vi "M300ShiftRun.vi"() -> ()   [LabVIEW 2012]
uses:
  <vilib>/Utility/miscctls.llb/LVDateTimeRec.ctl
panel:
  out "array":string[][](array[string])
  out "date string 2":string
  out "EndTime 3":string
  out "EndTime 2":string
  out "Numeric":i32
  out "date string 3":string
  out "©]1-4":dbl
  out "©]1-3":dbl
  out "早1-1":dbl
  out "©]1-1":dbl
  out "©]1-2":dbl
  out "早1-2":dbl
  out "©]2":dbl
  out "早2":dbl
  out "©]1":dbl
  out "早1":dbl
  in  "stop":bool
  out "中2":dbl
  out "中班1":dbl
  out "Start":timestamp
  out "End":timestamp
  out "ShiftC":timestamp
  out "ShiftA":timestamp
  out "ShiftB":timestamp
  out "date string":string
  out "x/y":dbl
  out "date/time string 2":string
  out "date/time string":string
  in  "EndTime":string
  in  "EndDate":string
  in  "BegTime":string
  in  "BegDate":string
  in  "date time rec":T1
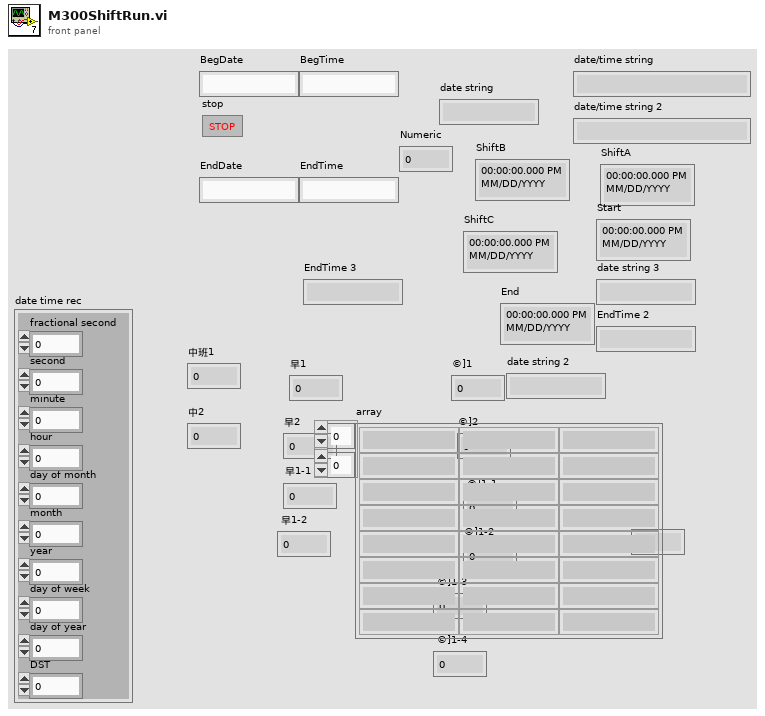
[diagram p1: front panel]
types:
  T1 = typedef "LVDateTimeRec.ctl" = cluster{"fractional second":dbl, "second":i32, "minute":i32, "hour":i32, "day of month":i32, "month":i32, "year":i32, "day of week":i32, "day of year":i32, "DST":i32}
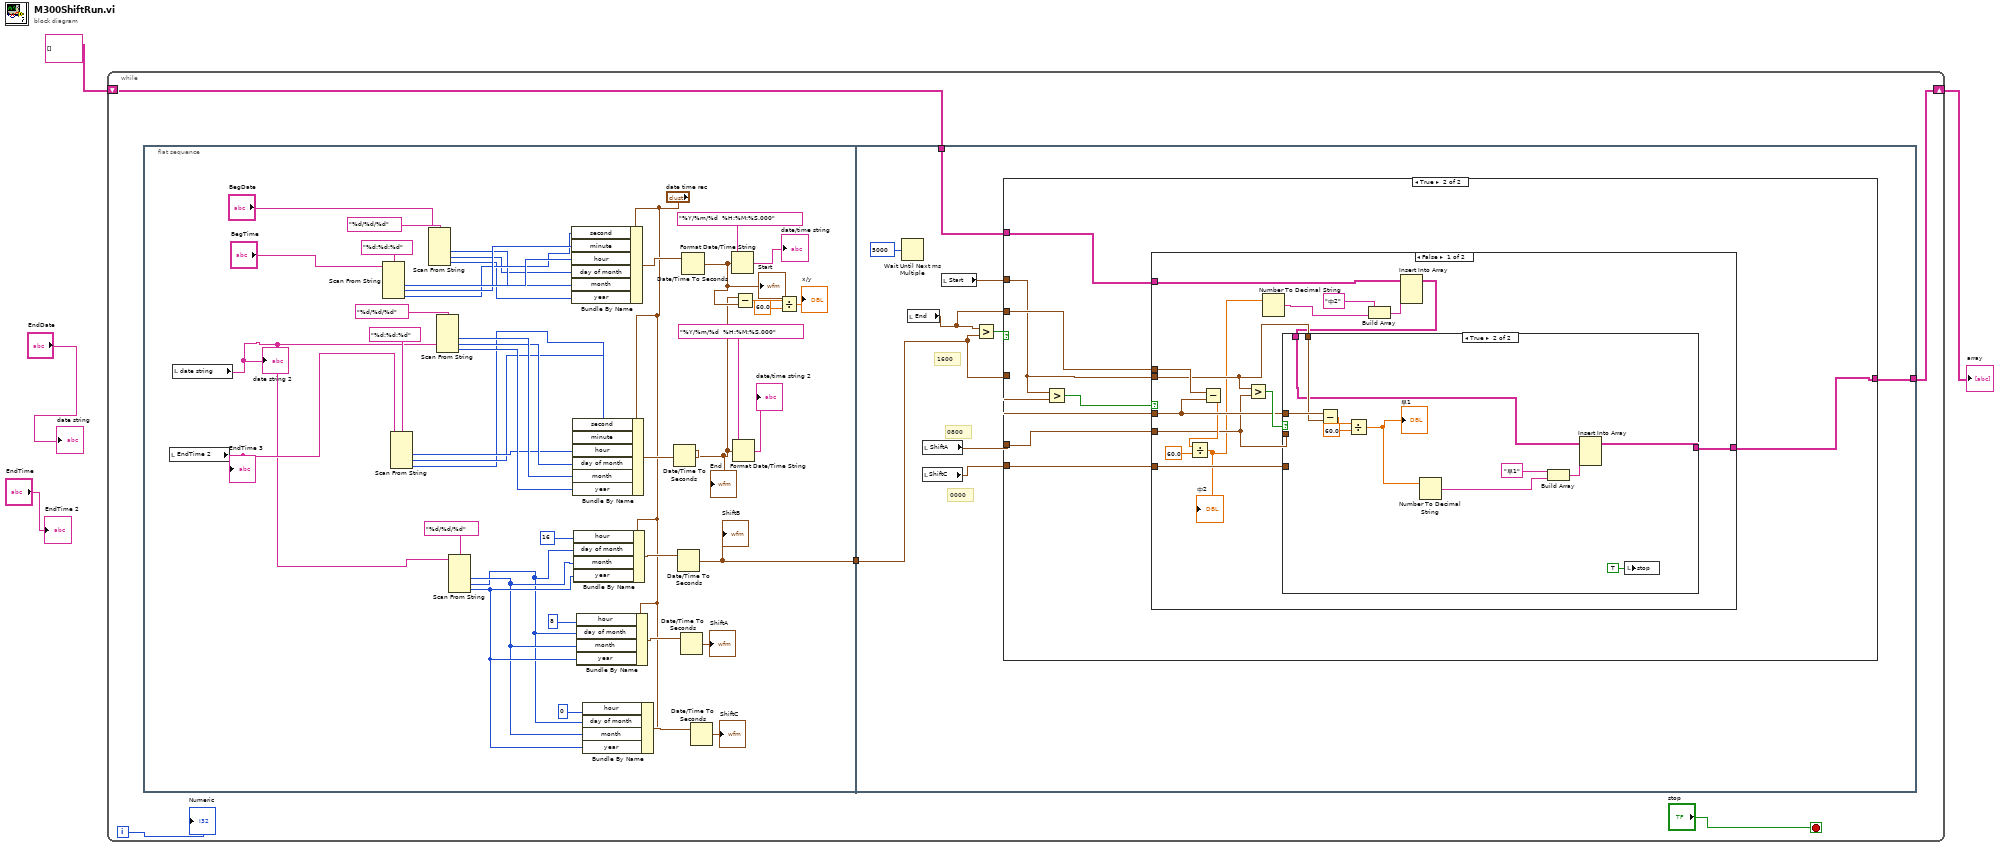
[diagram p0: block diagram]
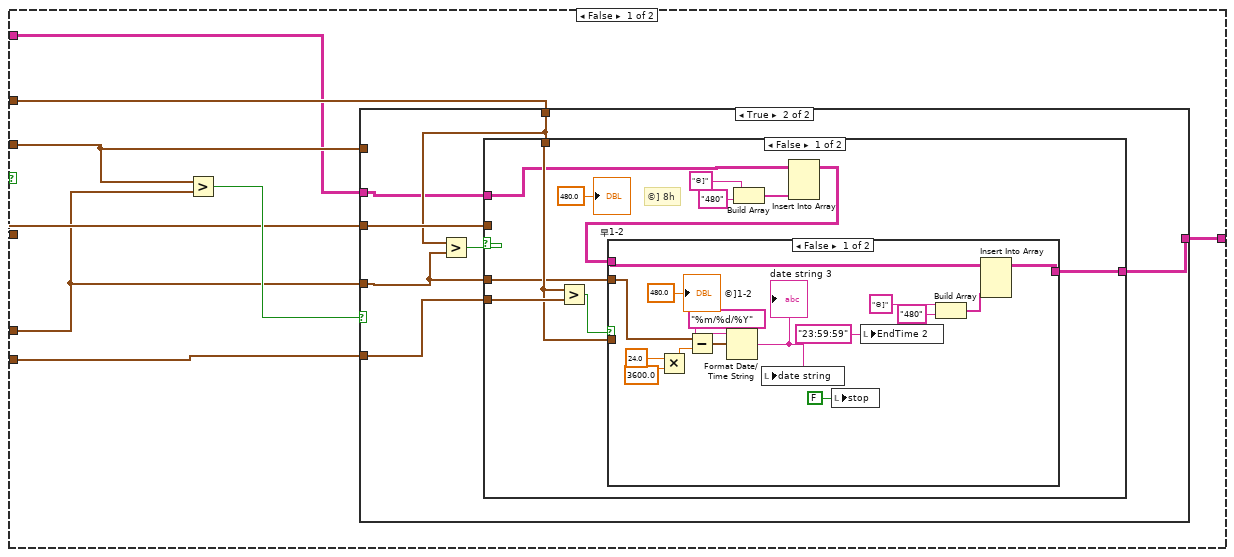
[diagram p2: hidden frame]
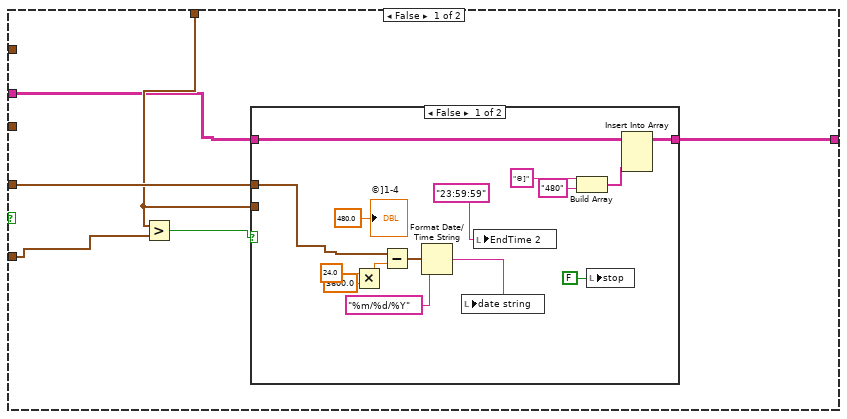
[diagram p3: hidden frame]
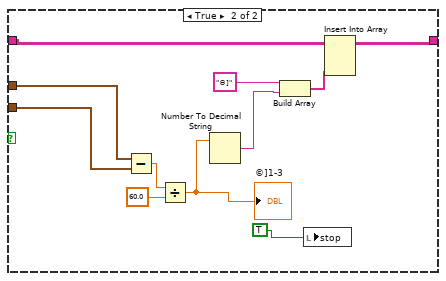
[diagram p4: hidden frame]
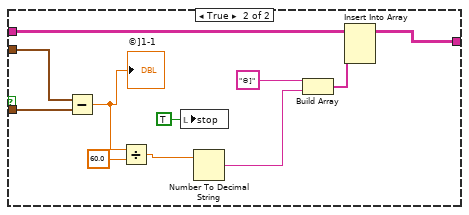
[diagram p5: hidden frame]
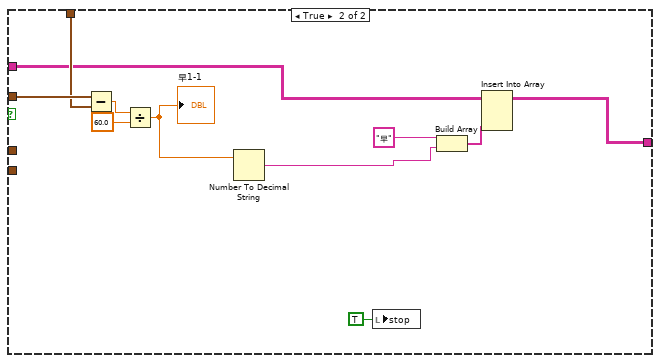
[diagram p6: hidden frame]
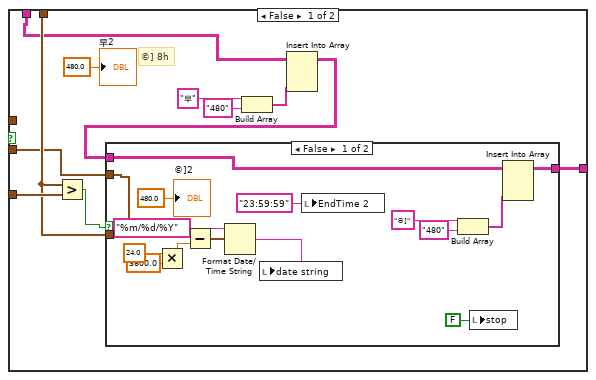
[diagram p7: hidden frame]
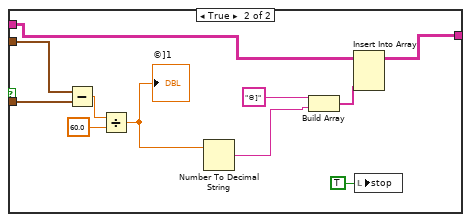
[diagram p8: hidden frame]
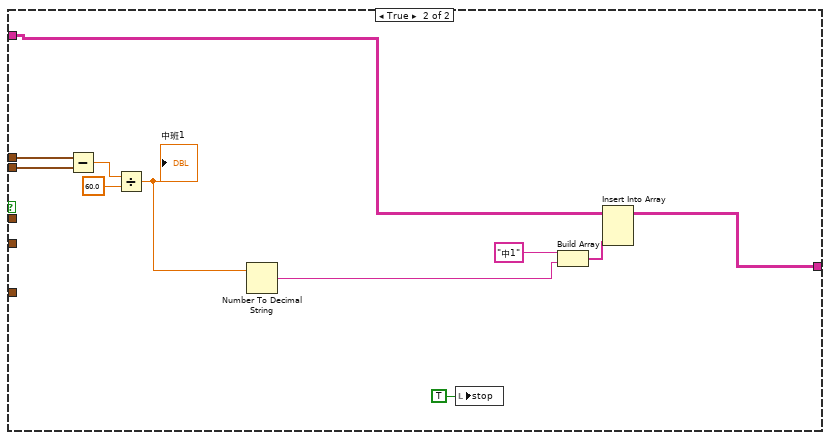
[diagram p9: hidden frame]
diagram:
  n1 = while {
    shift-right: [w6] -> w2
    shift-left: string[][] [] ("array") -> [w5]
    i -> [w8]
    stop <- "stop" stop-if-true
    n2 = flat-sequence {
      tunnel: [w11] -> w7
      tunnel: w7 -> [w58]
      tunnel: [w57] -> w6
      tunnel: w5 -> [w56]
      frame #0 {
        n3 = local read "EndTime 2"() -> (w12:string)
        "EndTime 3" <- w12
        n4 = local read "date string"() -> (w10:string)
        "date string 2" <- w10
        n5 = Scan From String(format string="%d:%d:%d", input string="BegTime") -> (output 1=w52:i32, output 2=w51:i32, output 3=w50:i32)  [unwired: 5 in, 3 out]
        n6 = Scan From String(format string="%d:%d:%d", input string=w12) -> (output 1=w44:i32, output 2=w43:i32, output 3=w42:i32)  [unwired: 5 in, 3 out]
        n7 = Scan From String(format string="%d/%d/%d", input string="BegDate") -> (output 1=w29:i32, output 2=w28:i32, output 3=w30:i32)  [unwired: 5 in, 3 out]
        n8 = Scan From String(format string="%d/%d/%d", input string=w10) -> (output 1=w47:i32, output 2=w46:i32, output 3=w45:i32)  [unwired: 5 in, 3 out]
        n9 = Scan From String(format string="%d/%d/%d", input string=w10) -> (output 1=w15:i32, output 2=w14:i32, output 3=w18:i32)  [unwired: 5 in, 3 out]
        n10 = Bundle By Name(cluster="date time rec", "second"=w50, "minute"=w51, "hour"=w52, "day of month"=w28, "month"=w29, "year"=w30) -> (w41:T1)
        n11 = Bundle By Name(cluster="date time rec", "second"=w42, "minute"=w43, "hour"=w44, "day of month"=w46, "month"=w47, "year"=w45) -> (w38:T1)
        n12 = Bundle By Name(cluster="date time rec", "hour"=16, "day of month"=w14, "month"=w15, "year"=w18) -> (w26:T1)
        n13 = Bundle By Name(cluster="date time rec", "hour"=8, "day of month"=w14, "month"=w15, "year"=w18) -> (w23:T1)
        n14 = Bundle By Name(cluster="date time rec", "hour"=0, "day of month"=w14, "month"=w15, "year"=w18) -> (w21:T1)
        n15 = Date/Time To Seconds(2:w38) -> (0:w13:timestamp)  [unwired: 1 in]
        "End" <- w13
        n16 = Date/Time To Seconds(2:w26) -> (0:w11:timestamp)  [unwired: 1 in]
        "ShiftB" <- w11
        n17 = Date/Time To Seconds(2:w23) -> (0:→"ShiftA":timestamp)  [unwired: 1 in]
        n18 = Date/Time To Seconds(2:w41) -> (0:w25:timestamp)  [unwired: 1 in]
        "Start" <- w25
        n19 = Date/Time To Seconds(2:w21) -> (0:→"ShiftC":timestamp)  [unwired: 1 in]
        n20 = Format Date/Time String(time format string (%c)="%Y/%m/%d  %H:%M:%S.000", seconds (now)=w25) -> (date/time string=→"date/time string":string)  [unwired: 1 in]
        n21 = Format Date/Time String(time format string (%c)="%Y/%m/%d  %H:%M:%S.000", seconds (now)=w13) -> (date/time string=→"date/time string 2":string)  [unwired: 1 in]
        n22 = Subtract(x=w13, y=w25) -> (x-y=w37:dbl)
        n23 = Divide(x=w37, y=60.0) -> (x/y=→"x/y":dbl)
      }
      frame #1 {
        # "0000"
        # "0800"
        # "1600"
        n24 = Wait Until Next ms Multiple(millisecond multiple=u32 5000) -> ()  [unwired: 1 out]
        n25 = local read "End"() -> (w60:timestamp)
        n26 = local read "ShiftC"() -> (w62:timestamp)
        n27 = local read "ShiftA"() -> (w61:timestamp)
        n28 = local read "Start"() -> (w63:timestamp)
        n29 = Greater?(x=w60, y=w58) -> (0:w59:bool)
        n30 = case shown="True" w59 {
          tunnel: w58 -> [w69 w164]
          tunnel: w60 -> [w70 w166]
          tunnel: w61 -> [w67 w163]
          tunnel: w62 -> [w68 w162]
          tunnel: w63 -> [w66 w161]
          tunnel: w56 -> [w65 w160]
          tunnel: [w64 w159] -> w57
          frame False {
            n31 = Greater?(x=w70, y=w67) -> (0:w71:bool)
            n32 = case shown="True" w71 {
              tunnel: w70 -> [_ _]
              tunnel: w69 -> [_ w110]
              tunnel: w68 -> [w76 w109]
              tunnel: w67 -> [w77 w107]
              tunnel: w66 -> [w74 w106]
              tunnel: w65 -> [w73 w105]
              tunnel: [w72 w104] -> w64
              frame False {
                n33 = Greater?(x=w74, y=w76) -> (0:w75:bool)
                n34 = case shown="False" w75 {
                  tunnel: w77 -> [w87 w103]
                  tunnel: w74 -> [_ w102]
                  tunnel: [w79 w96] -> w72
                  tunnel: w73 -> [w78 w95]
                  frame False {
                    n35 = Multiply(x=24.0, y=3600.0) -> (x*y=w92:dbl)
                    n36 = Subtract(x=w87, y=w92) -> (x-y=w89:timestamp)
                    n37 = Format Date/Time String(time format string (%c)="%m/%d/%Y", seconds (now)=w89) -> (date/time string=w86:string)  [unwired: 1 in]
                    n38 = local write "date string"(w86) -> ()
                    n39 = local write "EndTime 2"("23:59:59") -> ()
                    n40 = Build Array("©]", "480" ("element")) -> (w80:string[])
                    n41 = local write "stop"(FALSE ("stop")) -> ()
                    n42 = Insert Into Array(array=w78, new element=w80) -> (w79:string[][])  [unwired: 2 in]
                    "©]1-4" <- 480.0 ("Numeric")
                  }
                  frame True {
                    n43 = Subtract(x=w103, y=w102) -> (x-y=w100:dbl)
                    n44 = Divide(x=w100, y=60.0) -> (x/y=w94:dbl)
                    "©]1-3" <- w94
                    n45 = Number To Decimal String(number=w94) -> (decimal integer string=w93:string)  [unwired: 1 in]
                    n46 = Build Array("©]", w93) -> (w97:string[])
                    n47 = local write "stop"(TRUE ("stop")) -> ()
                    n48 = Insert Into Array(array=w95, new element=w97) -> (w96:string[][])  [unwired: 2 in]
                  }
                }
              }
              frame True {
                n49 = Greater?(x=w106, y=w107) -> (0:w108:bool)
                n50 = case shown="False" w108 {
                  tunnel: w110 -> [_ w158]
                  tunnel: w106 -> [w119 w157]
                  tunnel: w109 -> [w121 _]
                  tunnel: w107 -> [w117 _]
                  tunnel: w105 -> [w113 w148]
                  tunnel: [w116 w151] -> w104
                  frame False {
                    # "©] 8h"
                    n51 = Greater?(x=w119, y=w121) -> (0:w120:bool)
                    n52 = Build Array("©]", "480" ("element")) -> (w114:string[])
                    n53 = Insert Into Array(array=w113, new element=w114) -> (w111:string[][])  [unwired: 2 in]
                    n54 = case shown="False" w120 {
                      tunnel: w117 -> [w131 w147]
                      tunnel: w119 -> [_ w146]
                      tunnel: [w123 w138] -> w116
                      tunnel: w111 -> [w122 w137]
                      frame False {
                        n55 = Multiply(x=24.0, y=3600.0) -> (x*y=w136:dbl)
                        n56 = Subtract(x=w131, y=w136) -> (x-y=w133:timestamp)
                        n57 = Format Date/Time String(time format string (%c)="%m/%d/%Y", seconds (now)=w133) -> (date/time string=w128:string)  [unwired: 1 in]
                        "date string 3" <- w128
                        n58 = local write "date string"(w128) -> ()
                        n59 = local write "stop"(FALSE ("stop")) -> ()
                        n60 = local write "EndTime 2"("23:59:59" ("EndTime 2")) -> ()
                        n61 = Build Array("©]", "480" ("element")) -> (w125:string[])
                        n62 = Insert Into Array(array=w122, new element=w125) -> (w123:string[][])  [unwired: 2 in]
                        "©]1-2" <- 480.0 ("Numeric")
                      }
                      frame True {
                        n63 = Subtract(x=w147, y=w146) -> (x-y=w142:dbl)
                        "©]1-1" <- w142
                        n64 = Divide(x=w142, y=60.0) -> (x/y=w140:dbl)
                        n65 = local write "stop"(TRUE ("stop")) -> ()
                        n66 = Number To Decimal String(number=w140) -> (decimal integer string=w139:string)  [unwired: 1 in]
                        n67 = Build Array("©]", w139) -> (w143:string[])
                        n68 = Insert Into Array(array=w137, new element=w143) -> (w138:string[][])  [unwired: 2 in]
                      }
                    }
                    "早1-2" <- 480.0 ("Numeric")
                  }
                  frame True {
                    n69 = Subtract(x=w158, y=w157) -> (x-y=w155:dbl)
                    n70 = Divide(x=w155, y=60.0) -> (x/y=w149:dbl)
                    "早1-1" <- w149
                    n71 = Number To Decimal String(number=w149) -> (decimal integer string=w150:string)  [unwired: 1 in]
                    n72 = local write "stop"(TRUE ("stop")) -> ()
                    n73 = Build Array("早", w150) -> (w152:string[])
                    n74 = Insert Into Array(array=w148, new element=w152) -> (w151:string[][])  [unwired: 2 in]
                  }
                }
              }
            }
          }
          frame True {
            n75 = Greater?(x=w161, y=w164) -> (0:w165:bool)
            n76 = case shown="False" w165 {
              tunnel: w166 -> [w179 w240]
              tunnel: w161 -> [w175 w239]
              tunnel: w164 -> [w180 _]
              tunnel: w163 -> [w174 _]
              tunnel: w162 -> [w178 _]
              tunnel: w160 -> [w170 w230]
              tunnel: [w173 w233] -> w159
              frame False {
                n77 = Subtract(x=w179, y=w180) -> (x-y=w177:dbl)
                n78 = Divide(x=w177, y=60.0) -> (x/y=w169:dbl)
                "中2" <- w169
                n79 = Greater?(x=w175, y=w174) -> (0:w181:bool)
                n80 = Number To Decimal String(number=w169) -> (decimal integer string=w168:string)  [unwired: 1 in]
                n81 = Build Array("中2", w168) -> (w171:string[])
                n82 = Insert Into Array(array=w170, new element=w171) -> (w167:string[][])  [unwired: 2 in]
                n83 = case shown="True" w181 {
                  tunnel: w180 -> [_ w229]
                  tunnel: w175 -> [w190 w228]
                  tunnel: w178 -> [w192 _]
                  tunnel: w174 -> [w188 _]
                  tunnel: w167 -> [w183 w219]
                  tunnel: [w187 w222] -> w173
                  frame False {
                    # "©] 8h"
                    n84 = Greater?(x=w190, y=w192) -> (0:w191:bool)
                    n85 = Build Array("早", "480" ("element")) -> (w185:string[])
                    n86 = Insert Into Array(array=w183, new element=w185) -> (w182:string[][])  [unwired: 2 in]
                    n87 = case shown="False" w191 {
                      tunnel: w188 -> [w202 w218]
                      tunnel: w190 -> [_ w217]
                      tunnel: [w194 w211] -> w187
                      tunnel: w182 -> [w193 w208]
                      frame False {
                        n88 = Multiply(x=24.0, y=3600.0) -> (x*y=w207:dbl)
                        n89 = Subtract(x=w202, y=w207) -> (x-y=w204:timestamp)
                        n90 = Format Date/Time String(time format string (%c)="%m/%d/%Y", seconds (now)=w204) -> (date/time string=w200:string)  [unwired: 1 in]
                        n91 = local write "date string"(w200) -> ()
                        n92 = local write "EndTime 2"("23:59:59" ("EndTime 2")) -> ()
                        n93 = Build Array("©]", "480" ("element")) -> (w196:string[])
                        n94 = local write "stop"(FALSE ("stop")) -> ()
                        n95 = Insert Into Array(array=w193, new element=w196) -> (w194:string[][])  [unwired: 2 in]
                        "©]2" <- 480.0 ("Numeric")
                      }
                      frame True {
                        n96 = Subtract(x=w218, y=w217) -> (x-y=w215:dbl)
                        n97 = Divide(x=w215, y=60.0) -> (x/y=w210:dbl)
                        "©]1" <- w210
                        n98 = Number To Decimal String(number=w210) -> (decimal integer string=w209:string)  [unwired: 1 in]
                        n99 = Build Array("©]", w209) -> (w212:string[])
                        n100 = Insert Into Array(array=w208, new element=w212) -> (w211:string[][])  [unwired: 2 in]
                        n101 = local write "stop"(TRUE ("stop")) -> ()
                      }
                    }
                    "早2" <- 480.0 ("Numeric")
                  }
                  frame True {
                    n102 = Subtract(x=w229, y=w228) -> (x-y=w226:dbl)
                    n103 = Divide(x=w226, y=60.0) -> (x/y=w221:dbl)
                    "早1" <- w221
                    n104 = Number To Decimal String(number=w221) -> (decimal integer string=w220:string)  [unwired: 1 in]
                    n105 = Build Array("早1", w220) -> (w223:string[])
                    n106 = Insert Into Array(array=w219, new element=w223) -> (w222:string[][])  [unwired: 2 in]
                    n107 = local write "stop"(TRUE ("stop")) -> ()
                  }
                }
              }
              frame True {
                n108 = Subtract(x=w240, y=w239) -> (x-y=w237:dbl)
                n109 = Divide(x=w237, y=60.0) -> (x/y=w232:dbl)
                "中班1" <- w232
                n110 = Number To Decimal String(number=w232) -> (decimal integer string=w231:string)  [unwired: 1 in]
                n111 = local write "stop"(TRUE ("stop")) -> ()
                n112 = Build Array("中1", w231) -> (w234:string[])
                n113 = Insert Into Array(array=w230, new element=w234) -> (w233:string[][])  [unwired: 2 in]
              }
            }
          }
        }
      }
    }
    "Numeric" <- w8
  }
  "array" <- w2
  "date string" <- "EndDate"
  "EndTime 2" <- "EndTime"
